vi "Error Dialogue - Out of Range.vi"(7 "Parameter Name":string, 8 "error in":errorcluster, 9 "Range":T1, 10 "Parameter Value":dbl, 11 "Parameter Units":string) -> (0 "error out":errorcluster)   [LabVIEW 2015, in "Utility.lvlib"]
doc: "Displays a dialogue indicating the desired parameter is out of range."
uses:
  Utility.lvlib
  Typedef/Range.ctl
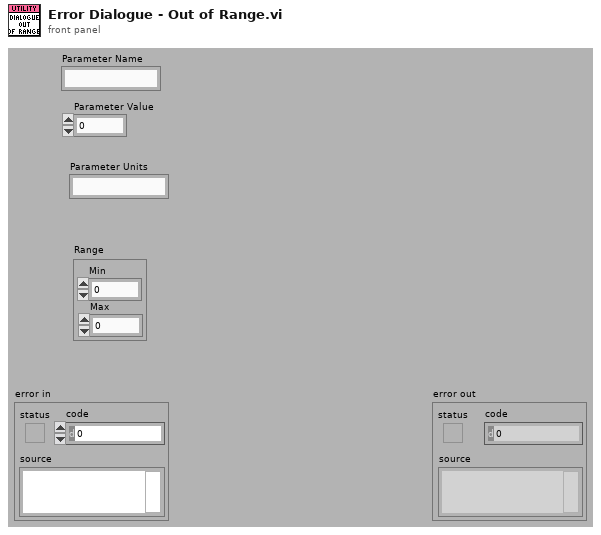
[diagram p1: front panel]
types:
  T1 = typedef "Utility.lvlib/Range.ctl" = cluster{"Min":dbl, "Max":dbl}
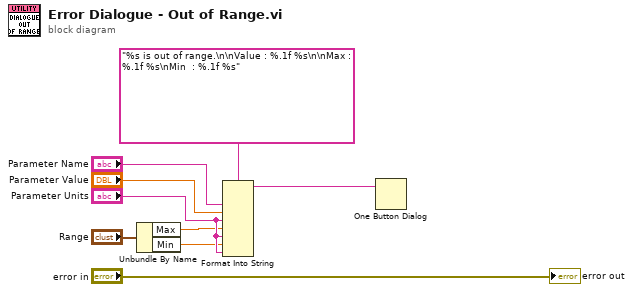
[diagram p0: block diagram]
diagram:
  n1 = Unbundle By Name("Range") -> ("Max"=w3:dbl, "Min"=w2:dbl)
  n2 = Format Into String(format string="%s is out of range.\n\nValue : %.1f %s\n\nMax : %.1f %s\nMin  : %.1f %s", "Parameter Name", "Parameter Value", "Parameter Units", w3, "Parameter Units", w2, "Parameter Units") -> (resulting string=w1:string)  [unwired: 2 in, 1 out]
  n3 = One Button Dialog(message=w1) -> ()  [unwired: 1 in, 1 out]
  "error out" <- "error in"
